vi "Open file in ImageJ.vi"(8 "Process Index":i32, 11 "Current File Num":i32) -> ()   [LabVIEW 2013]
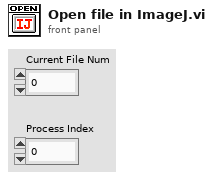
[diagram p1: front panel]
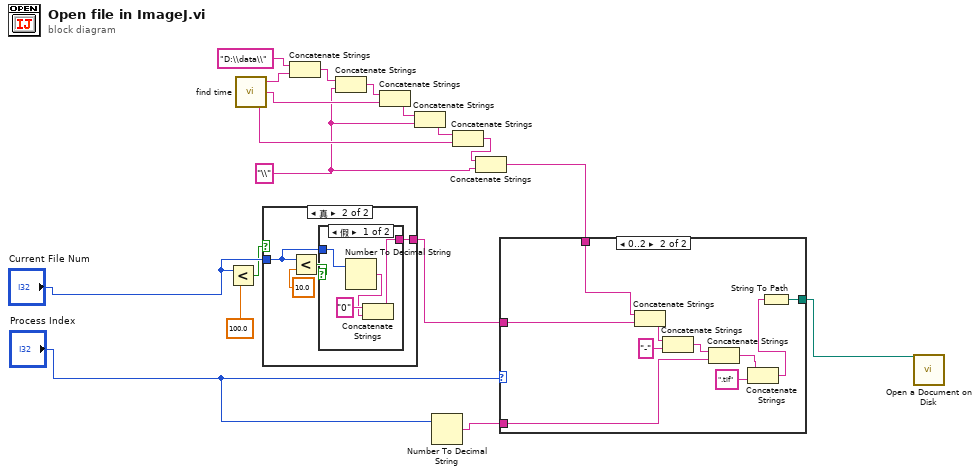
[diagram p0: block diagram]
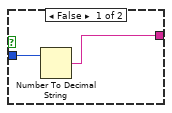
[diagram p2: hidden frame]
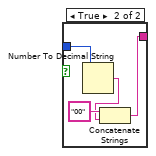
[diagram p3: hidden frame]
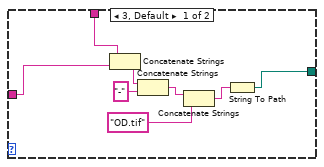
[diagram p4: hidden frame]
diagram:
  w7 = "\\" ("字符串")
  n1 = Less?(x="Current File Num", y=100.0) -> (x < y?=w4:bool)
  n2 = call "find time.vi"() -> ("day"=w9:string, "month"=w12:string, "year"=w15:string)  [unwired: 3 in]
  n3 = case shown="真" w4 {
    tunnel: "Current File Num" -> [w20 w22]
    tunnel: [w19 w21] -> w3
    frame False {
      n4 = Number To Decimal String(number=w20) -> (decimal integer string=w19:string)  [unwired: 1 in]
    }
    frame True {
      n5 = Less?(x=w22, y=10.0) -> (x < y?=w23:bool)
      n6 = case shown="假" w23 {
        tunnel: w22 -> [w27 w32]
        tunnel: [w25 w29] -> w21
        frame False {
          n7 = Number To Decimal String(number=w27) -> (decimal integer string=w26:string)  [unwired: 1 in]
          n8 = Concatenate Strings("0" ("字符串"), w26) -> (w25:string)
        }
        frame True {
          n9 = Number To Decimal String(number=w32) -> (decimal integer string=w30:string)  [unwired: 1 in]
          n10 = Concatenate Strings("00" ("字符串"), w30) -> (w29:string)
        }
      }
    }
  }
  n11 = Concatenate Strings("D:\\data\\", w15) -> (w14:string)
  n12 = Concatenate Strings(w14, w7) -> (w13:string)
  n13 = Concatenate Strings(w13, w12) -> (w11:string)
  n14 = Concatenate Strings(w11, w7) -> (w10:string)
  n15 = Number To Decimal String(number="Process Index") -> (decimal integer string=w6:string)  [unwired: 1 in]
  n16 = Concatenate Strings(w10, w9) -> (w8:string)
  n17 = Concatenate Strings(w8, w7) -> (w2:string)
  n18 = case shown="0..2" "Process Index" {
    tunnel: [w34 w50] -> w1
    tunnel: w3 -> [w37 w49]
    tunnel: w6 -> [_ w45]
    tunnel: w2 -> [w33 w44]
    frame 3, Default {
      n19 = Concatenate Strings(w33, w37) -> (w40:string)
      n20 = Concatenate Strings(w40, "-" ("字符串")) -> (w38:string)
      n21 = Concatenate Strings(w38, "OD.tif" ("字符串")) -> (w35:string)
      n22 = String To Path(string=w35) -> (path=w34:path)
    }
    frame 0..2 {
      n23 = Concatenate Strings(w44, w49) -> (w48:string)
      n24 = Concatenate Strings(w48, "-" ("字符串")) -> (w46:string)
      n25 = Concatenate Strings(w46, w45) -> (w42:string)
      n26 = Concatenate Strings(w42, ".tif" ("字符串")) -> (w41:string)
      n27 = String To Path(string=w41) -> (path=w50:path)
    }
  }
  n28 = call <vilib>:"Open a Document on Disk.vi"("document path"=w1) -> ()  [unwired: 6 in, 1 out]
